vi "GetRAndT.vi"(7 "Track":string="47.302", 8 "TIn":string, 9 "RIn":string, 10 "Raw":i32, 11 "Item Names":string[](array[string])) -> (2 "T":string, 3 "R":string)   [LabVIEW 2014]
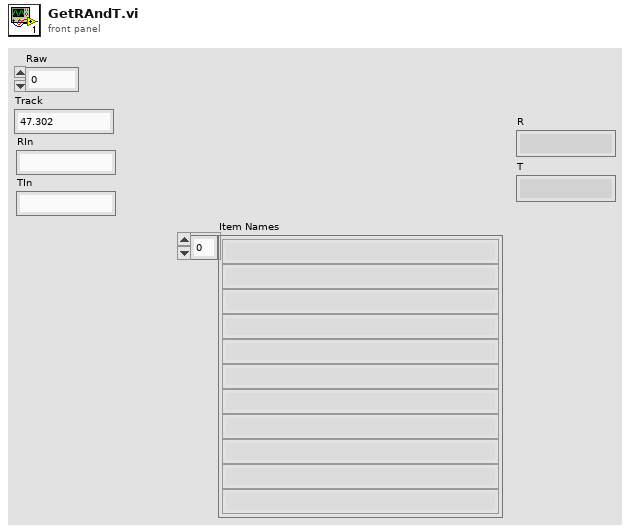
[diagram p1: front panel]
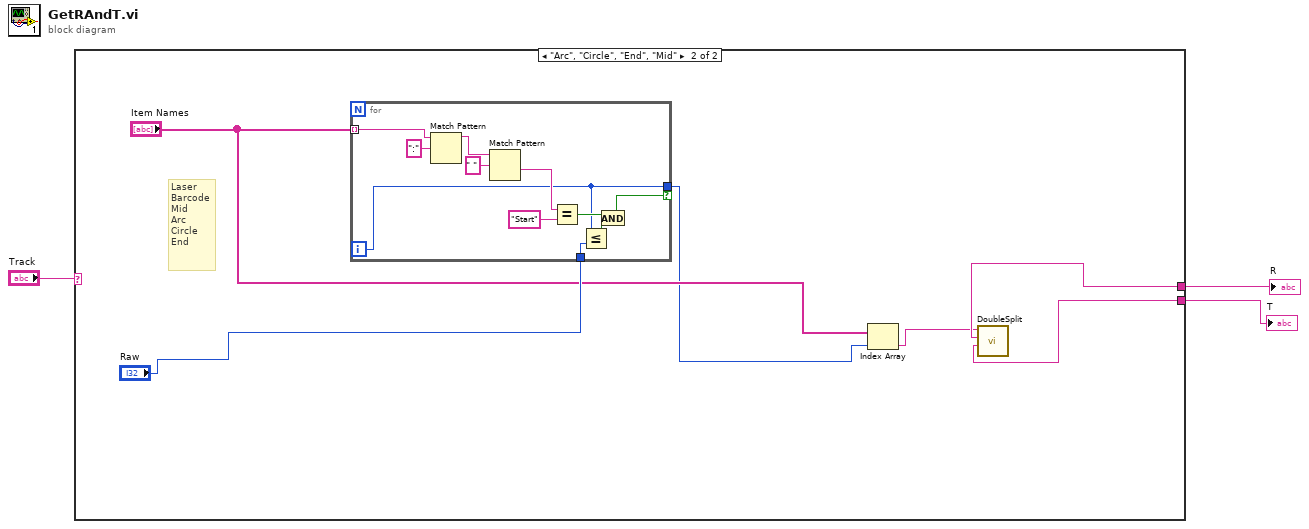
[diagram p0: block diagram]
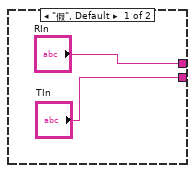
[diagram p2: hidden frame]
diagram:
  n1 = case shown="\"Arc\", \"Circle\", \"End\", \"Mid\"" "Track" {
    tunnel: ["RIn" w8] -> w3
    tunnel: ["TIn" w7] -> w2
    frame "假", Default {
    }
    frame "Arc", "Circle", "End", "Mid" {
      # "Laser\nBarcode\nMid\nArc\nCircle\nEnd"
      n2 = for {
        tunnel: "Item Names" -> [w22] mode=indexing
        tunnel: [w15] -> w9 if=w13
        tunnel: "Raw" -> [w14]
        i -> [w15]
        n3 = Match Pattern(string=w22, regular expression=":" ("正则表达式")) -> (before substring=w20:string)  [unwired: 1 in, 3 out]
        n4 = Match Pattern(string=w20, regular expression=" " ("正则表达式")) -> (after substring=w18:string)  [unwired: 1 in, 3 out]
        n5 = Equal?(x=w18, y="Start") -> (x = y?=w16:bool)
        n6 = Less Or Equal?(x=w15, y=w14) -> (x <= y?=w12:bool)
        n7 = And(x=w16, y=w12) -> (x .and. y?=w13:bool)
      }
      n8 = Index Array(array="Item Names", index=w9) -> (element=w6:string)
      n9 = call "DoubleSplit.vi"("Track"=w6) -> ("T"=w7:string, "R"=w8:string)  [unwired: 9 out]
    }
  }
  "R" <- w3
  "T" <- w2
